vi "Flatten Debug Cluster to String.vi"(8 "error in (no error)":errorcluster) -> (0 "error out":errorcluster, 3 "Flattened Cluster":string)   [LabVIEW 2009]
uses:
  Actions for FG's.ctl
  Debug Shared/Debug Data Packet.ctl
  TypeDefs/State Machine/Main State.ctl
  Status Indicators.ctl
  TypeDefs/Sensor TypeDefs/GPS Data.ctl
  TypeDefs/Sensor TypeDefs/SICK Array.ctl
  Remote Control/Motor Command.ctl
  TypeDefs/Queue TypeDefs/Motor Instruction.ctl
  TypeDefs/Queue TypeDefs/Motor State.ctl
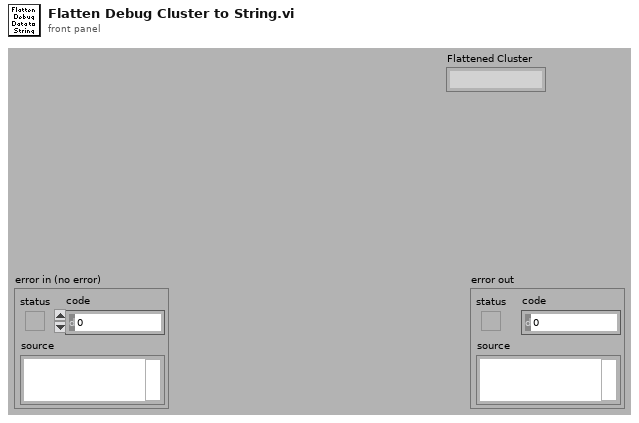
[diagram p1: front panel]
types:
  T1 = typedef "Status Indicators.ctl" = cluster{"GPS Init Complete":bool, "SICK Init Complete":bool, "Compass Init Complete":bool, "Camera Init Complete":bool, "Sensors Init Complete":bool, "Motors Init Complete":bool, "MC Heartbeat":bool, "Motors On?":bool, "Encoders Zeroed?":bool, "JAUS Go":bool}
  T2 = typedef "Debug Data Packet.ctl" = cluster{"Main State out":T3, "HB out":bool, "Status Indicators out":T1, "RC/!Run out":bool, "AUT/!NAV":bool, "Compass Data":dbl, "GPS Data":T4, "SICK Data":T5, "Target Bearing":dbl, "Target Sector":i16, "Calculated sector":i16, "RC Command":T6, "Motor Loop Instruction":T7, "Waypoints reached":i8, "Battery Voltage":dbl, "Local Pose":cluster{"X Coordinate":dbl, "Y Coordinate":dbl}, "EVS HB":bool}
  T3 = typedef "Main State.ctl" = enum16{"Startup", "Wait for Init", "Initialize Sensors", "Wait for Saftey Disable", "Check Saftey", "Wait for GO", "Run", "Remote Control", "Stop"}
  T4 = typedef "GPS Data.ctl" = cluster{"Latitude":dbl, "Longitude":dbl}
  T5 = typedef "SICK Array.ctl" = u16[]
  T6 = typedef "Motor Command.ctl" = cluster{"Speed":i16, "Turn":i16}
  T7 = typedef "Motor Instruction.ctl" = cluster{"Motor State":T8, "Motor Command":T6}
  T8 = typedef "Motor State.ctl" = enum16{"Wait", "Initialize", "Check FET", "Run", "Stop"}
  T9 = typedef "Actions for FG's.ctl" = enum16{"Read", "Write"}
  T10 = typedef "LocalPose.ctl" = cluster{" X":dbl, " Y":dbl, " Z":dbl, "Position RMS":dbl, "Roll":dbl, "Pitch":dbl, "Yaw":dbl, "Attitude RMS":dbl, "TimeRec":T11}
  T11 = typedef "TimeRec.ctl" = cluster{"Milliseconds":u32, "Seconds":u32, "Minutes":u32, "Hours":u32, "Day":u32}
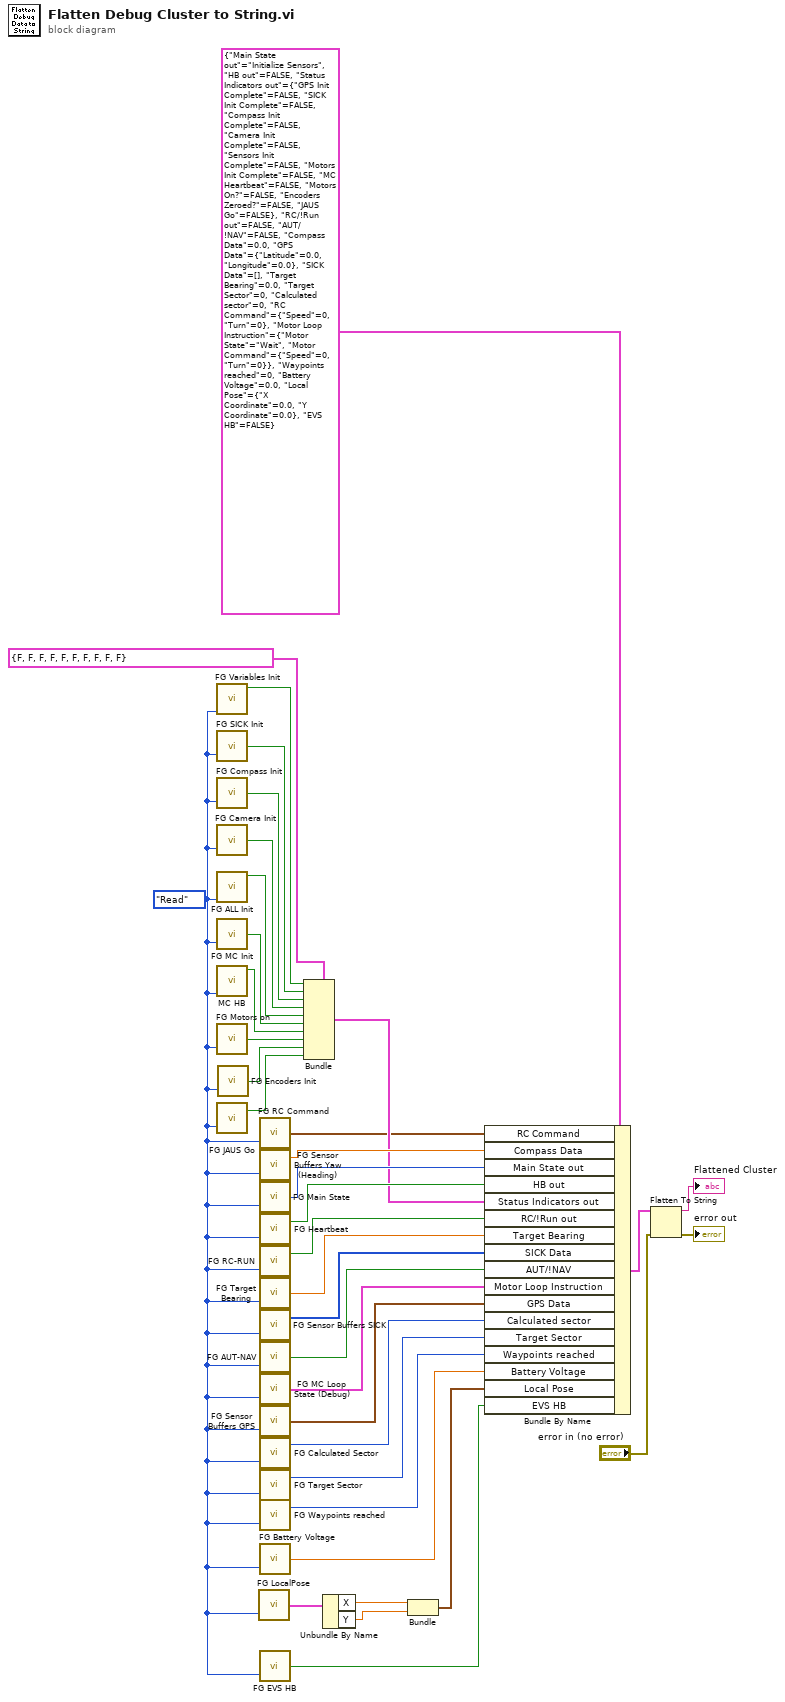
[diagram p0: block diagram]
diagram:
  w2 = Actions_for_FG's."Read" ("FG Action")
  n1 = call "FG Variables Init.vi"("FG Action"=w2) -> ("Variables Init out"=w16:bool)  [unwired: 10 in]
  n2 = call "FG SICK Init.vi"("FG Action"=w2) -> ("SICK Init out"=w22:bool)  [unwired: 1 in]
  n3 = call "FG Compass Init.vi"("FG Action"=w2) -> ("Compass Init out"=w21:bool)  [unwired: 1 in]
  n4 = call "FG Camera Init.vi"("FG Action"=w2) -> ("Camera Init out"=w20:bool)  [unwired: 1 in]
  n5 = call "FG ALL Init.vi"("FG Action"=w2) -> ("ALL Init out"=w9:bool)  [unwired: 10 in]
  n6 = call "FG MC Init.vi"("FG Action"=w2) -> ("MC Init out"=w19:bool)  [unwired: 1 in]
  n7 = call "MC HB.vi"("FG Action"=w2) -> ("MC HB out"=w18:bool)  [unwired: 10 in]
  n8 = call "FG Motors on.vi"("FG Action"=w2) -> ("Motors on ? out"=w17:bool)  [unwired: 1 in]
  n9 = call "FG JAUS Go.vi"("FG Action (Read)"=w2) -> ("Go Out"=w7:bool)  [unwired: 1 in]
  n10 = call "FG Encoders Init.vi"("FG Action"=w2) -> ("Encoders  Zeroed out"=w8:bool)  [unwired: 1 in]
  n11 = call "FG LocalPose.vi"("FG Action (Read)"=w2) -> ("LocalPose out"=w6:T10)  [unwired: 1 in]
  n12 = call "FG RC Command.vi"("FG Action"=w2) -> ("Motor Command out"=w26:T6)  [unwired: 1 in]
  n13 = call "FG Sensor Buffers Yaw (Heading).vi"("FG Action (Read)"=w2) -> ("Yaw Buffer Out"=w37:dbl)  [unwired: 2 in]
  n14 = call "FG Main State.vi"("FG Action"=w2) -> ("Main State out"=w36:T3)  [unwired: 1 in]
  n15 = call "FG Heartbeat.vi"("FG Action"=w2) -> ("HB out"=w35:bool)  [unwired: 2 in]
  n16 = call "FG RC-RUN.vi"("FG Action (Read)"=w2) -> ("RC/!Run out"=w33:bool)  [unwired: 2 in]
  n17 = call "FG Target Bearing.vi"("FG Action (Read)"=w2) -> ("Target Bearing out"=w28:dbl)  [unwired: 1 in]
  n18 = call "FG Sensor Buffers SICK.vi"("FG Actions (Read)"=w2) -> ("SICK Buffer out"=w27:T5)  [unwired: 2 in]
  n19 = call "FG AUT-NAV.vi"("FG Action (Read)"=w2) -> ("Aut/!Nav out"=w14:bool)  [unwired: 1 in]
  n20 = call "FG MC Loop State (Debug).vi"("FG Action (Read)"=w2) -> ("Motor Instruction out"=w24:T7)  [unwired: 1 in]
  n21 = call "FG Sensor Buffers GPS.vi"("FG Action (Read)"=w2) -> ("GPS Buffer out"=w15:T4)  [unwired: 1 in]
  n22 = call "FG Calculated Sector.vi"("FG Action (Read)"=w2) -> ("Target sector out"=w13:i16)  [unwired: 2 in]
  n23 = call "FG Target Sector.vi"("FG Action (Read)"=w2) -> ("Target sector out"=w12:i16)  [unwired: 2 in]
  n24 = call "FG Waypoints reached.vi"("FG Action (Read)"=w2) -> ("Waypoints reached out"=w11:i8)  [unwired: 2 in]
  n25 = call "FG Battery Voltage.vi"("FG Action"=w2) -> ("Battery Voltage out"=w10:dbl)  [unwired: 1 in]
  n26 = call "FG EVS HB.vi"("FG Action"=w2) -> ("EVS HB Out"=w1:bool)  [unwired: 1 in]
  n27 = Bundle(cluster=T1 {"GPS Init Complete"=FALSE, "SICK Init Complete"=FALSE, "Compass Init Complete"=FALSE, "Camera Init Complete"=FALSE, "Sensors Init Complete"=FALSE, "Motors Init Complete"=FALSE, "MC Heartbeat"=FALSE, "Motors On?"=FALSE, "Encoders Zeroed?"=FALSE, "JAUS Go"=FALSE} ("Status Indicators in"), "GPS Init Complete"=w16, "SICK Init Complete"=w22, "Compass Init Complete"=w21, "Camera Init Complete"=w20, "Sensors Init Complete"=w9, "Motors Init Complete"=w19, "MC Heartbeat"=w18, "Motors On?"=w17, "Encoders Zeroed?"=w8, "JAUS Go"=w7) -> (w34:T1)
  n28 = Unbundle By Name(w6) -> ("X"=w5:dbl, "Y"=w4:dbl)
  n29 = Bundle("X"=w5, "Y"=w4) -> (w3:cluster{" X":dbl, " Y":dbl})  [unwired: 1 in]
  n30 = Bundle By Name(cluster=T2 {"Main State out"=enum."Initialize Sensors", "HB out"=FALSE, "Status Indicators out"={"GPS Init Complete"=FALSE, "SICK Init Complete"=FALSE, "Compass Init Complete"=FALSE, "Camera Init Complete"=FALSE, "Sensors Init Complete"=FALSE, "Motors Init Complete"=FALSE, "MC Heartbeat"=FALSE, "Motors On?"=FALSE, "Encoders Zeroed?"=FALSE, "JAUS Go"=FALSE}, "RC/!Run out"=FALSE, "AUT/!NAV"=FALSE, "Compass Data"=0.0, "GPS Data"={"Latitude"=0.0, "Longitude"=0.0}, "SICK Data"=[], "Target Bearing"=0.0, "Target Sector"=0, "Calculated sector"=0, "RC Command"={"Speed"=0, "Turn"=0}, "Motor Loop Instruction"={"Motor State"=enum."Wait", "Motor Command"={"Speed"=0, "Turn"=0}}, "Waypoints reached"=0, "Battery Voltage"=0.0, "Local Pose"={"X Coordinate"=0.0, "Y Coordinate"=0.0}, "EVS HB"=FALSE} ("Cluster"), "RC Command"=w26, "Compass Data"=w37, "Main State out"=w36, "HB out"=w35, "Status Indicators out"=w34, "RC/!Run out"=w33, "Target Bearing"=w28, "SICK Data"=w27, "AUT/!NAV"=w14, "Motor Loop Instruction"=w24, "GPS Data"=w15, "Calculated sector"=w13, "Target Sector"=w12, "Waypoints reached"=w11, "Battery Voltage"=w10, "Local Pose"=w3, "EVS HB"=w1) -> (w32:T2)
  n31 = Flatten To String(anything=w32, error in (no error)="error in (no error)") -> (data string=→"Flattened Cluster":string, error out=→"error out":errorcluster)  [unwired: 2 in, 1 out]
